vi "subCustomMergerError.vi"(11 "Errors":errorcluster[](array[cluster])) -> (3 "error out":errorcluster)   [LabVIEW 2020, in "CommonHelpers.lvlib"]
uses:
  CommonHelpers.lvlib
  <vilib>/Utility/error.llb/whitespace.ctl
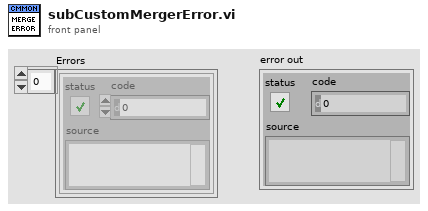
[diagram p1: front panel]
types:
  T1 = typedef "whitespace.ctl" = u16
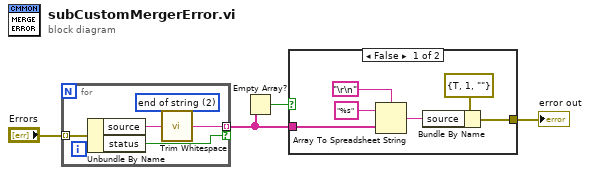
[diagram p0: block diagram]
diagram:
  n1 = for {
    tunnel: "Errors" -> [w9] mode=indexing
    tunnel: [w6] -> w2 mode=indexing if=w7
    w5 = T1 2 items=["both", "start of string", "end of string"] ("location (both)")
    n2 = Unbundle By Name(w9) -> ("source"=w8:string, "status"=w7:bool)
    n3 = call <vilib>:"Trim Whitespace.vi"("string"=w8, "location (both)"=w5) -> ("trimmed string"=w6:string)
  }
  n4 = Empty Array?(array=w2) -> (empty?=w1:bool)
  n5 = case shown="False" w1 {
    tunnel: w2 -> [w13 _]
    tunnel: [w11 _] -> w3
    frame False {
      n6 = Array To Spreadsheet String(delimiter (Tab)="\r\n", array=w13, 3:"%s" ("format string")) -> (spreadsheet string=w12:string)
      n7 = Bundle By Name(cluster=errorcluster {"status"=TRUE, "code"=1, "source"=""} ("error out"), "source"=w12) -> (w11:errorcluster)
    }
    frame True {
    }
  }
  "error out" <- w3
